vi "TTB Write.vi"(4 "error in":errorcluster, 6 "TTB Cluster In":cluster{i32, u16, i16, i16}, 7 "refnum in":refnum<file>) -> (0 "error out":errorcluster, 3 "refnum out":refnum<file>)   [LabVIEW 2011]
doc: "TTB Write.vi\n\nThis VI writes a single time table cluster to the time table file (.TTB). The program parses the TTB cluster to its four parts, swaps the bits (to be compliant with the C++ version) and saves the information to the time table file."
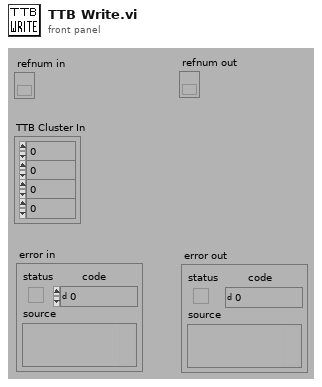
[diagram p1: front panel]
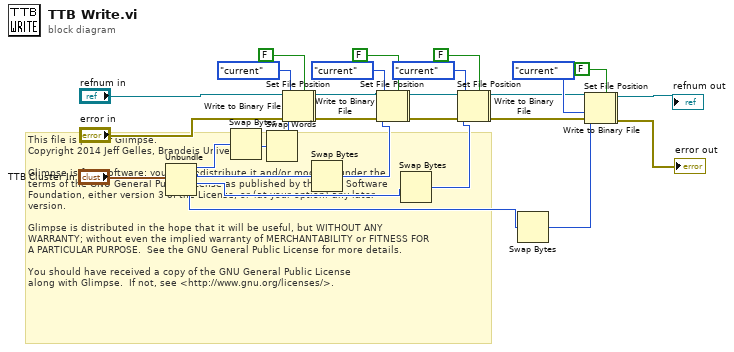
[diagram p0: block diagram]
diagram:
  # "This file is part of Glimpse. \nCopyright 2014 Jeff Gelles, Brandeis University.    \n\nGlimpse is free software: you can redistribute it and/or modify it under the \nterms of the GNU General Public License as published by the Free Software \nFoundation, either version 3 of the License, or (at your option) any later \nversion.\n\nGlimpse is distributed in the hope that it will be useful, but WITHOUT ANY \nWARRANTY; without even the implied warranty of MERCHANTABILITY or FITNESS FOR \nA PARTICULAR PURPOSE.  See the GNU General Public License for more details.\n\nYou should have received a copy of the GNU General Public License\nalong with Glimpse.  If not, see <http://www.gnu.org/licenses/>."
  n1 = Unbundle("TTB Cluster In") -> (w28:i32, w27:u16, w24:i16, w35:i16)
  n2 = Swap Bytes(anything=w28) -> (byte swapped=w30:i32)
  n3 = Swap Words(1:w30) -> (0:w29:i32)
  n4 = Set File Position(refnum="refnum in", from (0:start)=enum16{"start", "end", "current"}."current" ("pos mode (0:2)"), error in="error in") -> (refnum out=w3:refnum<file>, error out=w2:errorcluster)  [unwired: 1 out]
  n5 = Write to Binary File(file (use dialog)=w3, data=w29, error in=w2, 5:FALSE ("prepend array or string size? (T)")) -> (refnum out=w19:refnum<file>, error out=w16:errorcluster)  [unwired: 3 out]
  n6 = Swap Bytes(anything=w27) -> (byte swapped=w25:u16)
  n7 = Set File Position(refnum=w19, from (0:start)=enum16{"start", "end", "current"}."current" ("pos mode (0:2)"), error in=w16) -> (refnum out=w6:refnum<file>, error out=w5:errorcluster)  [unwired: 1 out]
  n8 = Write to Binary File(file (use dialog)=w6, data=w25, error in=w5, 5:FALSE ("prepend array or string size? (T)")) -> (refnum out=w18:refnum<file>, error out=w15:errorcluster)  [unwired: 3 out]
  n9 = Swap Bytes(anything=w24) -> (byte swapped=w22:i16)
  n10 = Set File Position(refnum=w18, from (0:start)=enum16{"start", "end", "current"}."current" ("pos mode (0:2)"), error in=w15) -> (refnum out=w9:refnum<file>, error out=w8:errorcluster)  [unwired: 1 out]
  n11 = Write to Binary File(file (use dialog)=w9, data=w22, error in=w8, 5:FALSE ("prepend array or string size? (T)")) -> (refnum out=w17:refnum<file>, error out=w14:errorcluster)  [unwired: 3 out]
  n12 = Swap Bytes(anything=w35) -> (byte swapped=w20:i16)
  n13 = Set File Position(refnum=w17, from (0:start)=enum16{"start", "end", "current"}."current" ("pos mode (0:2)"), error in=w14) -> (refnum out=w12:refnum<file>, error out=w11:errorcluster)  [unwired: 1 out]
  n14 = Write to Binary File(file (use dialog)=w12, data=w20, error in=w11, 5:FALSE ("prepend array or string size? (T)")) -> (refnum out=→"refnum out":refnum<file>, error out=→"error out":errorcluster)  [unwired: 3 out]
